vi "writetotexttest.vi"() -> ()   [LabVIEW 2018]
uses:
  <vilib>/Utility/file.llb/Write Delimited Spreadsheet (I64).vi
panel:
  in  "file path (dialog if empty)":path
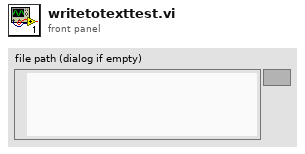
[diagram p1: front panel]
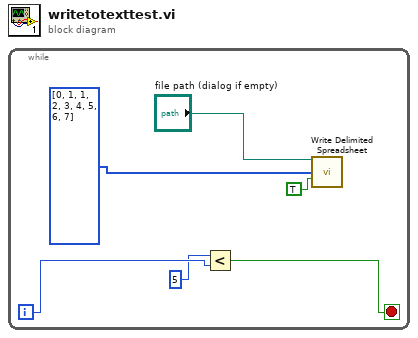
[diagram p0: block diagram]
diagram:
  n1 = while {
    i -> [w2]
    stop <- w4 stop-if-true
    n2 = Less?(x=5, y=w2) -> (x < y?=w4:bool)
    n3 = call-poly <vilib>:"Write Delimited Spreadsheet.vi"("file path (dialog if empty)"="file path (dialog if empty)", "1D data"=i32[] [0, 1, 1, 2, 3, 4, 5, 6, 7], "append to file? (new file:F)"=TRUE) -> ()  [unwired: 11 in, 2 out]
  }
